vi "Temperature (SubVI).vi"(8 "Input Array":variant[](array[variant]), 11 "JSON string":string) -> (0 "output array":variant[](array[variant]))   [LabVIEW 2017]
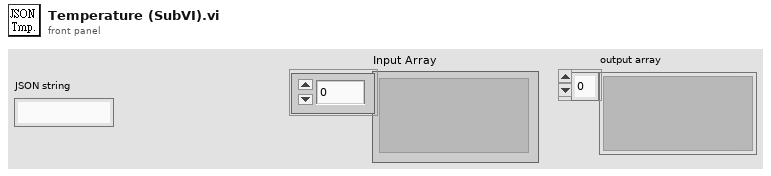
[diagram p1: front panel]
types:
  T1 = cluster{"LTargetTemp":dbl, "LTemp":dbl[], "RTargetTemp":dbl, "RTemp":dbl[]}
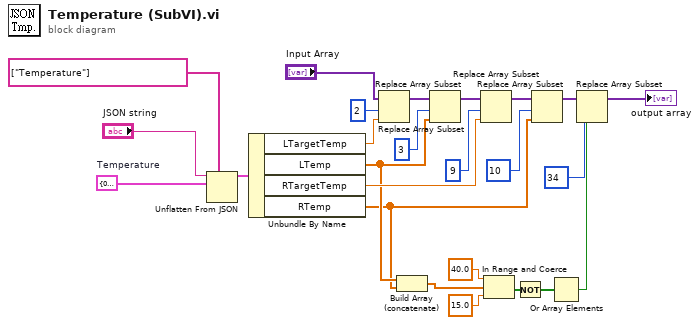
[diagram p0: block diagram]
diagram:
  w23 = T1 {"LTargetTemp"=0.0, "LTemp"=[26.2, 26.6, 25.9, 24.9, 25.5, 25.6], "RTargetTemp"=0.0, "RTemp"=[26.3, 26.3, 26.3, 26.3, 28.0, 27.5]}  # Temperature
  n1 = Unflatten From JSON(path=string[] ["Temperature"], JSON string="JSON string", type and defaults=w23) -> (value=w22:T1)  [unwired: 4 in, 1 out]
  n2 = Unbundle By Name(w22) -> ("LTargetTemp"=w19:dbl, "LTemp"=w8:dbl[], "RTargetTemp"=w14:dbl, "RTemp"=w7:dbl[])
  n3 = Replace Array Subset(array="Input Array", new element=w19, index=2) -> (w17:variant[])
  n4 = Build Array (concatenate)(w8, w7) -> (w6:dbl[])
  n5 = Replace Array Subset(array=w17, new element=w8, index=3) -> (w15:variant[])
  n6 = Replace Array Subset(array=w15, new element=w14, index=9) -> (w12:variant[])
  n7 = In Range and Coerce(upper limit=40.0, x=w6, lower limit=15.0) -> (In Range?=w5:bool[])  [unwired: 1 out]
  n8 = Not(x=w5) -> (.not. x?=w1:bool[])
  n9 = Replace Array Subset(array=w12, new element=w7, index=10) -> (w11:variant[])
  n10 = Or Array Elements(Boolean array=w1) -> (logical OR=w3:bool)
  n11 = Replace Array Subset(array=w11, new element=w3, index=34) -> (→"output array":variant[])
